vi "Return Hardware Reference.vi"(8 "error in":errorcluster, 10 "System Hardware Reference":refnum<k20>, 11 "Controller in":refnum<class "Controller.lvclass">) -> (0 "error out":errorcluster, 3 "Controller out":refnum<class "Controller.lvclass">)   [LabVIEW 2016, in "SMI.lvlib" / "Controller.lvclass"]
uses:
  Controller.lvclass
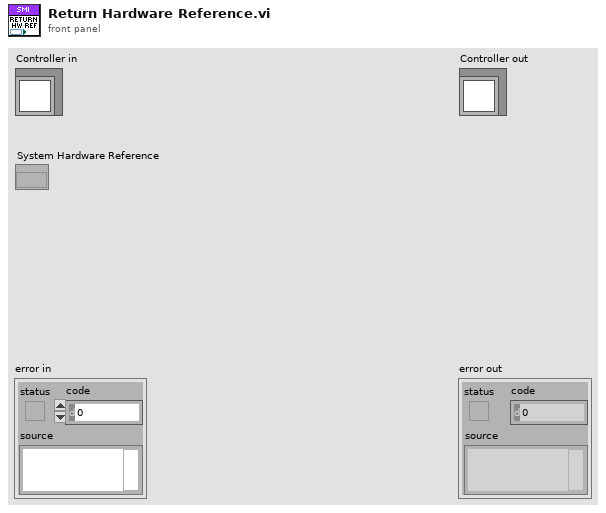
[diagram p1: front panel]
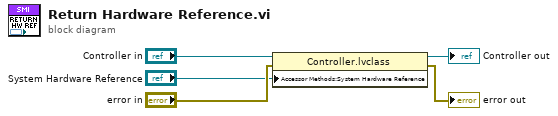
[diagram p0: block diagram]
diagram:
  n1 = property class="Controller.lvclass"(reference="Controller in", error in="error in", "Accessor Methods:System Hardware Reference"="System Hardware Reference") -> (reference out=→"Controller out":refnum<class "Controller.lvclass">, error out=→"error out":errorcluster)
